vi "SCM File Producer.vi"(3 "Source File":path=path "C:/ScopeBinaryData.bin", 4 "error in (no error)":errorcluster, 5 "# Channels":i32, 6 "Samples per Channel":i32, 7 "Data Queue":refnum<queue>) -> (0 "error out":errorcluster)   [LabVIEW 2013]
uses:
  ExecutionControlGlobal.vi
panel:
  out "Loop Time (ms)":dbl
  in  "Signal Selector":bool[](array[boolean])=[FALSE, TRUE, TRUE, TRUE, TRUE, TRUE, FALSE, FALSE]
  in  "Array":dbl[][](array[numeric])
  out "Data":dbl[][](graph)
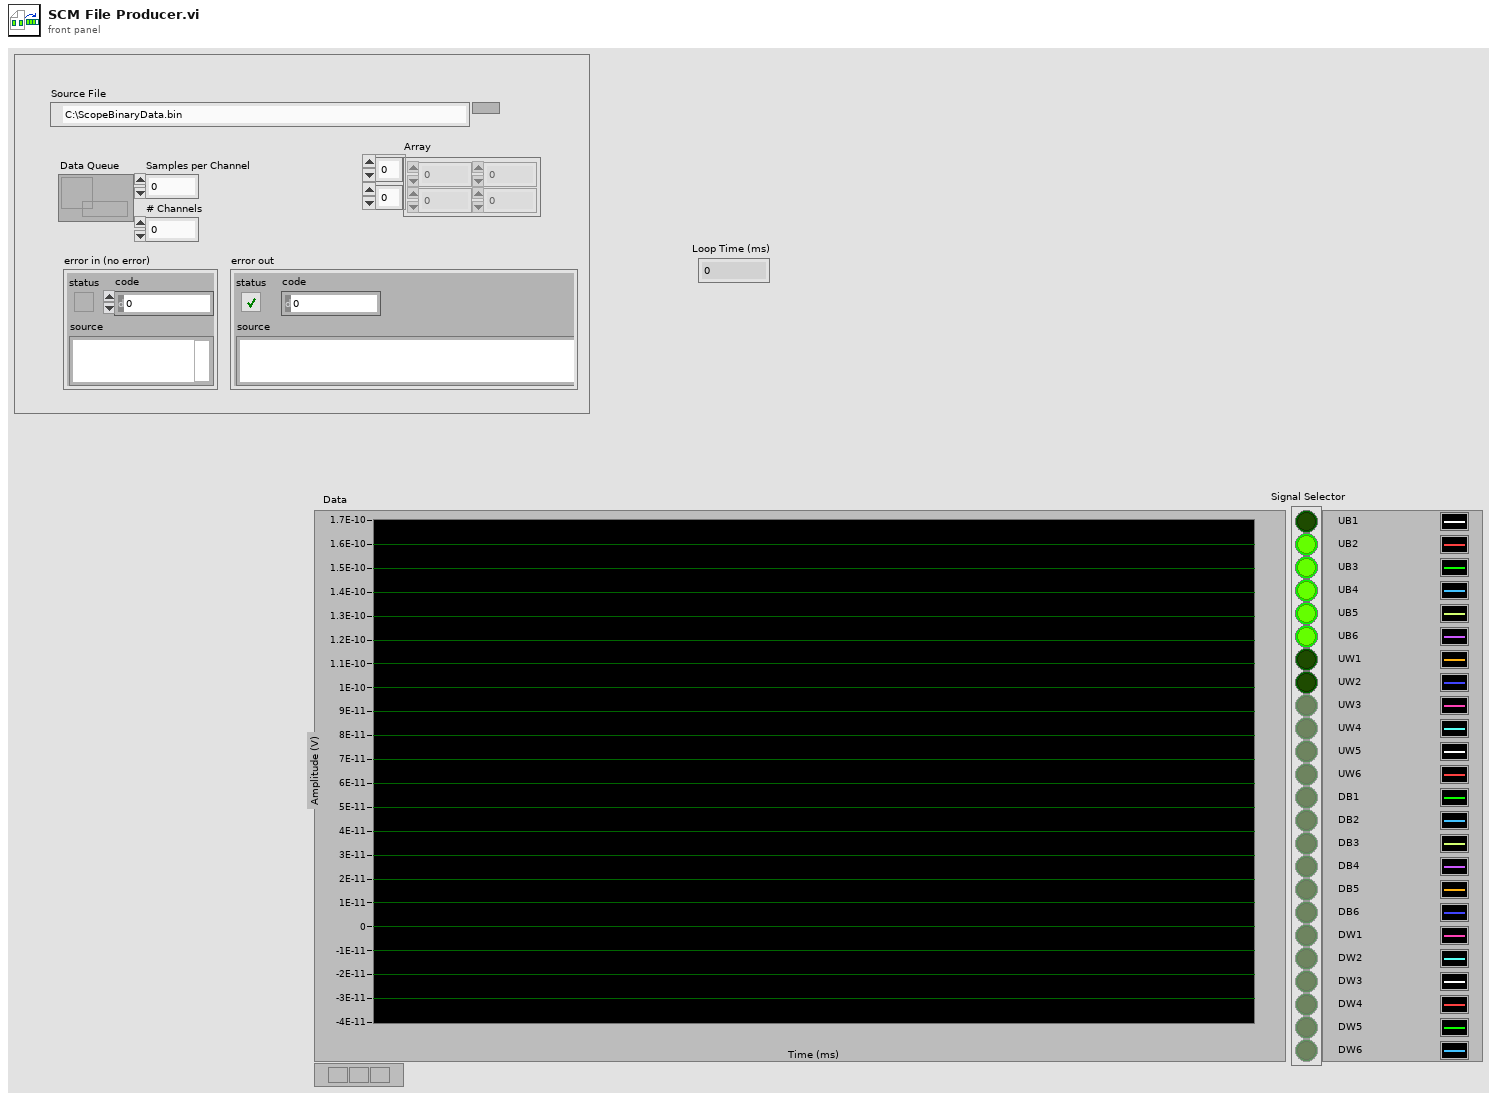
[diagram p1: front panel]
types:
  T1 = enum16{"open", "replace", "create", "open or create", "replace or create", "replace or create with confirmation"}
  T2 = enum16{"big-endian, network order", "native, host order", "little-endian"}
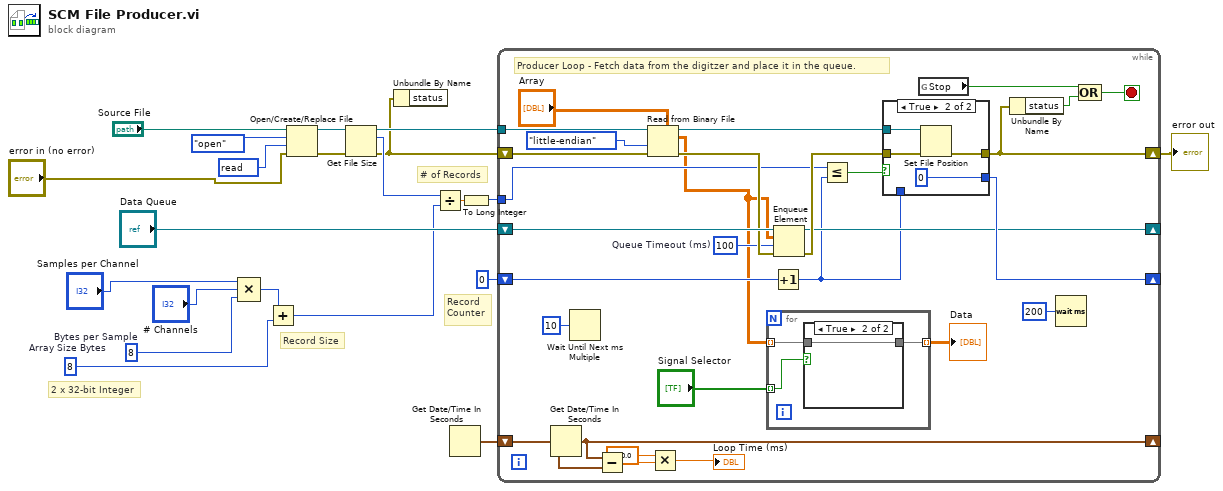
[diagram p0: block diagram]
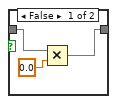
[diagram p2: hidden frame]
diagram:
  w13 = 8  # Array Size Bytes
  w12 = 8  # Bytes per Sample
  w4 = u32 2147483648 items=["read"=2147483648, "write"=1073741824, "read & write"=3221225472, "execute"=536870912, "all"=268435456] ("desired access (read & write)")
  # "# of Records"
  # "Record\nCounter"
  # "Record Size"
  # "2 x 32-bit Integer"
  n1 = Compound Arithmetic op=MULTIPLY("Samples per Channel", "# Channels", w12) -> (w11:i32)
  n2 = Add(x=w11, y=w13) -> (x+y=w10:i32)
  n3 = Open/Create/Replace File(file path (use dialog)="Source File", error in="error in (no error)", operation (0:open)=T1."open", access (0:read/write)=w4) -> (refnum out=w7:refnum<file>, error out=w8:errorcluster)  [unwired: 2 in, 1 out]
  n4 = Get File Size(file=w7, error in=w8) -> (refnum out=w21:refnum<file>, size (in bytes)=w20:i64, 0:w2:errorcluster)
  n5 = Unbundle By Name(w2) -> ()  [unwired: 1 out]
  n6 = Divide(x=w20, y=w10) -> (x/y=w19:dbl)
  n7 = Get Date/Time In Seconds() -> (seconds since 1Jan1904=w1:timestamp)
  n8 = To Long Integer(number=w19) -> (32bit integer=w18:i32)
  n9 = while {
    shift-right: [w46] -> w16
    shift-left: w2 -> [w47]
    tunnel: w21 -> [w48]
    shift-right: [w44] -> _
    shift-left: 0 -> [w32]
    tunnel: w18 -> [w34]
    shift-right: [w40] -> _
    shift-left: "Data Queue" -> [w43]
    shift-right: [w25] -> _
    shift-left: w1 -> [w26]
    stop <- w39 stop-if-true
    w37 = 100  # Queue Timeout (ms)
    # "Producer Loop - Fetch data from the digitzer and place it in the queue."
    n10 = Get Date/Time In Seconds() -> (seconds since 1Jan1904=w25:timestamp)
    n11 = Wait Until Next ms Multiple(millisecond multiple=u32 10) -> ()  [unwired: 1 out]
    n12 = Subtract(x=w25, y=w26) -> (x-y=w24:dbl)
    n13 = Read from Binary File(5:"Array", 8:w47, 9:T2."little-endian" ("byte order (0:big-endian, network order)"), 11:w48) -> (0:w42:errorcluster, 2:w28:dbl[][], 3:w45:refnum<file>)  [unwired: 2 in, 1 out]
    n14 = Multiply(x=1000.0, y=w24) -> (x*y=→"Loop Time (ms)":dbl)
    n15 = for {
      tunnel: "Signal Selector" -> [w53] mode=indexing
      tunnel: w28 -> [w52] mode=indexing
      tunnel: [w51] -> w27 mode=indexing
      n16 = case shown="True" w53 {
        tunnel: w52 -> [w56 w57]
        tunnel: [w54 w57] -> w51
        frame False {
          n17 = Multiply(x=w56, y=0.0) -> (x*y=w54:dbl[])
        }
        frame True {
        }
      }
    }
    "Data" <- w27
    n18 = Increment(x=w32) -> (x+1=w31:i32)
    n19 = Enqueue Element(queue=w43, element=w28, timeout in ms (-1)=w37, error in (no error)=w42) -> (queue out=w40:refnum<queue>, error out=w41:errorcluster)  [unwired: 1 out]
    n20 = Less Or Equal?(x=w34, y=w31) -> (x <= y?=w35:bool)
    n21 = case shown="True" w35 {
      tunnel: w41 -> [w59 w63]
      tunnel: [w59 w62] -> w46
      tunnel: w45 -> [_ w61]
      tunnel: [w58 0] -> w44
      tunnel: w31 -> [w58 _]
      frame False {
      }
      frame True {
        n22 = Set File Position(refnum=w61, error in=w63) -> (error out=w62:errorcluster)  [unwired: 2 in, 1 out]
      }
    }
    n23 = global read "ExecutionControlGlobal.vi" "Stop"() -> (w36:bool)
    n24 = Unbundle By Name(w46) -> ("status"=w49:bool)
    n25 = Wait (ms)(milliseconds to wait=u32 200) -> ()  [unwired: 1 out]
    n26 = Compound Arithmetic op=OR(w36, w49) -> (w39:bool)
  }
  "error out" <- w16
